vi "ROI entry-ROI MotorZ adjustment dialogue.vi"() -> (3 "Cancelled (Left button pressed)":bool)   [LabVIEW 2020]
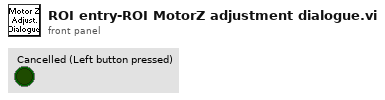
[diagram p1: front panel]
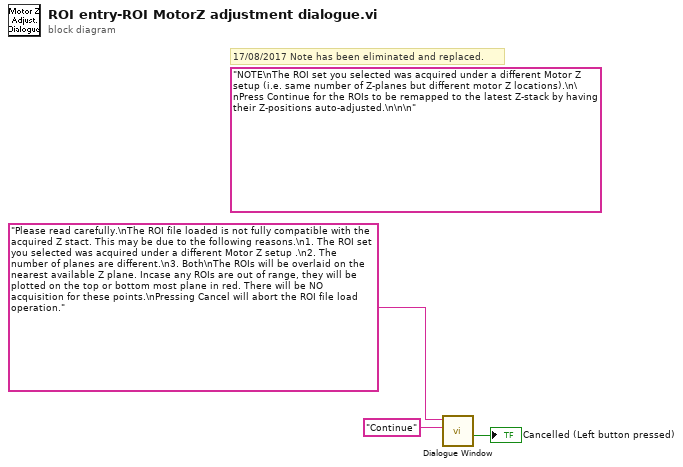
[diagram p0: block diagram]
diagram:
  (unwired) "NOTE\nThe ROI set you selected was acquired under a different Motor Z setup (i.e. same number of Z-planes but different motor Z locations).\n\nPress Continue for the ROIs to be remapped to the latest Z-stack by having their Z-positions auto-adjusted.\n\n\n" ("Message string")
  # "17/08/2017 Note has been eliminated and replaced."
  n1 = call "Dialogue Window.vi"("Caption-Right button (OK)"="Continue", "Message string"="Please read carefully.\nThe ROI file loaded is not fully compatible with the acquired Z stact. This may be due to the following reasons.\n1. The ROI set you selected was acquired under a different Motor Z setup .\n2. The number of planes are different.\n3. Both\nThe ROIs will be overlaid on the nearest available Z plane. Incase any ROIs are out of range, they will be plotted on the top or bottom most plane in red. There will be NO acquisition for these points.\nPressing Cancel will abort the ROI file load operation.") -> ("Cancelled (Left button pressed)"=→"Cancelled (Left button pressed)":bool)  [unwired: 7 in, 2 out]
